vi "getFilePattern.vi"(8 "error in (no error)":errorcluster, 11 "MS-Excel in":refnum<class "MS-Excel.lvclass">) -> (0 "error out":errorcluster, 1 "pattern":string, 2 "pattern label":string, 3 "MS-Excel out":refnum<class "MS-Excel.lvclass">)   [LabVIEW 2020, in "LabVIEW NPOI.lvlib" / "MS-Excel.lvclass"]
uses:
  MS-Excel.lvclass
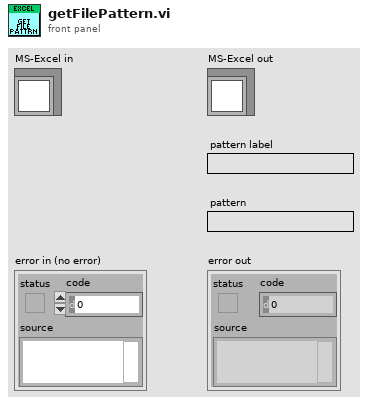
[diagram p1: front panel]
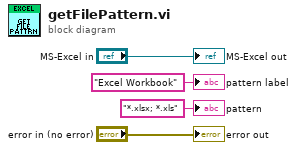
[diagram p0: block diagram]
diagram:
  "error out" <- "error in (no error)"
  "MS-Excel out" <- "MS-Excel in"
  "pattern" <- "*.xlsx; *.xls" ("pattern")
  "pattern label" <- "Excel Workbook" ("pattern label")
